vi "Run All.vi"(8 "Error In":errorcluster) -> (0 "Error Out":errorcluster)   [LabVIEW 2017, in "Tests.lvlib"]
uses:
  Tests.lvlib
  Version/Version.lvlib
  Writer/Writer.lvlib
  <vilib>/addons/_JKI Toolkits/Caraya/classes/Test/Test.lvclass
  Status/Status.lvlib
  To Msgpack/To Msgpack.lvlib
  Reader/Reader.lvlib
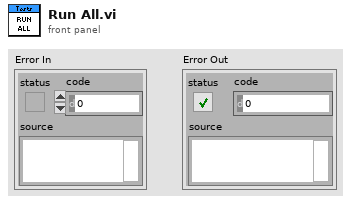
[diagram p1: front panel]
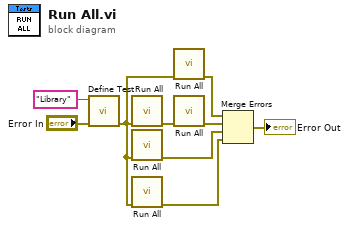
[diagram p0: block diagram]
diagram:
  n1 = call <vilib>:"Define Test.vi"("error in (no error)"="Error In", "Label (VI Title)"="Library") -> ("error out"=w2:errorcluster)  [unwired: 9 in]
  n2 = call "Run All.vi"("Error In"=w2) -> ("Error Out"=w4:errorcluster)  [unwired: 10 in]
  n3 = call "Run All.vi"("Error In"=w2) -> ("Error Out"=w5:errorcluster)  [unwired: 10 in]
  n4 = call "Run All.vi"("Error In"=w2) -> ("Error Out"=w1:errorcluster)  [unwired: 10 in]
  n5 = call "Run All.vi"("Error In"=w2) -> ("Error Out"=w9:errorcluster)  [unwired: 10 in]
  n6 = call "Run All.vi"("Error In"=w4) -> ("Error Out"=w3:errorcluster)  [unwired: 10 in]
  n7 = Merge Errors(w9, w3, w5, w1) -> (→"Error Out":errorcluster)
